vi "HW initialize hardware command.vi"(8 "error in (no error)":errorcluster, 10 "mode":T1, 11 "mmWave instrument in":refnum<class "mmWave instrument.lvclass">) -> (0 "error out":errorcluster, 3 "mmWave instrument out":refnum<class "mmWave instrument.lvclass">)   [LabVIEW 2019, in "HW Control.lvlib"]
uses:
  HW Control.lvlib
  SubVIs/mmWave instrument_class/mmWave instrument.lvclass
  SubVIs/mmWave instrument_class/Instrument mode.ctl
  SubVIs/mmWave instrument_class/Instrument state.ctl
  <vilib>/event_ctls.llb/usereventprio.ctl
  HW GV.vi
  Log/Log.lvlib
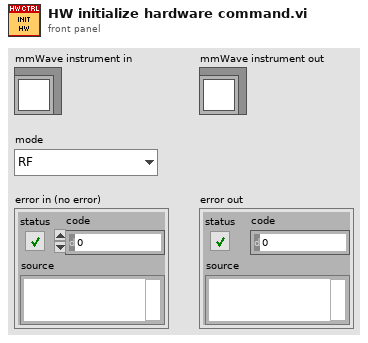
[diagram p1: front panel]
types:
  T1 = typedef "mmWave instrument.lvclass/Instrument mode.ctl" = enum16{"RF", "IF", "BB"}
  T2 = typedef "mmWave instrument.lvclass/Instrument state.ctl" = enum16{"Off", "Initialization", "Configuration", "Running", "Calibration"}
  T3 = typedef "usereventprio.ctl" = enum32{"high priority", "normal priority"}
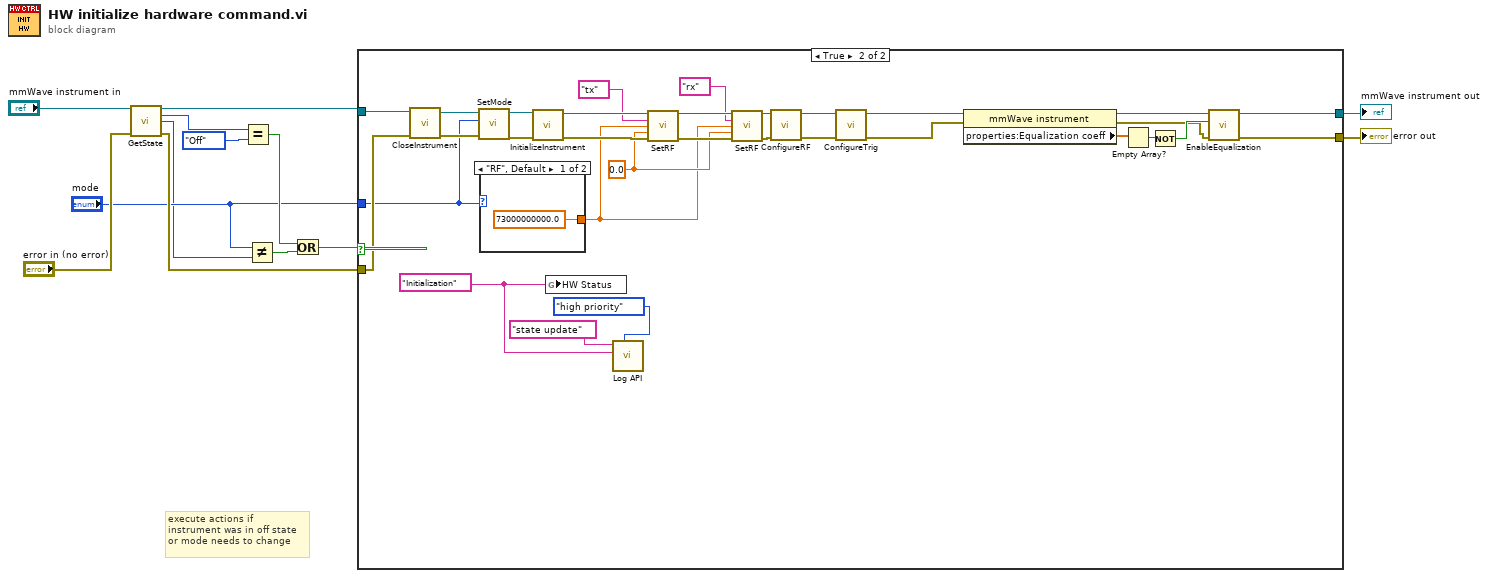
[diagram p0: block diagram]
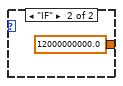
[diagram p3: hidden frame]
diagram:
  # "execute actions if\ninstrument was in off state\nor mode needs to change"
  n1 = call-dynamic "GetState.vi"("reference in"="mmWave instrument in", "error in (no error)"="error in (no error)") -> ("reference out"=w9:refnum<class "mmWave instrument.lvclass">, "state"=w2:T2, "mode"=w4:T1, "error out"=w11:errorcluster)  [unwired: 9 in, 1 out]
  n2 = Equal?(x=w2, y=Instrument_state."Off" ("x")) -> (x = y?=w7:bool)
  n3 = Not Equal?(x="mode", y=w4) -> (x != y?=w6:bool)
  n4 = Or(x=w7, y=w6) -> (x .or. y?=w8:bool)
  n5 = case shown="True" w8 {
    tunnel: w11 -> [w15 w40]
    tunnel: [w15 w20] -> w12
    tunnel: w9 -> [w14 w39]
    tunnel: "mode" -> [_ w27]
    tunnel: [w14 w25] -> w13
    frame False {
      # "no change needed"
    }
    frame True {
      w33 = 0.0 ("Gain")
      w38 = "Initialization" ("HW Status")
      n6 = call-dynamic "CloseInstrument.vi"("error in (no error)"=w40, "reference in"=w39) -> ("error out"=w45:errorcluster, "reference out"=w46:refnum<class "mmWave instrument.lvclass">)  [unwired: 8 in]
      n7 = call-dynamic "SetMode.vi"("error in (no error)"=w45, "instr mode"=w27, "reference in"=w46) -> ("error out"=w44:errorcluster, "reference out"=w43:refnum<class "mmWave instrument.lvclass">)  [unwired: 7 in]
      n8 = case shown="\"RF\", Default" w27 {
        tunnel: [73000000000.0 ("Frequency") 12000000000.0 ("Frequency")] -> w32
        frame "RF", Default {
        }
        frame "IF" {
        }
      }
      n9 = call-dynamic "InitializeInstrument.vi"("error in (no error)"=w44, "reference in"=w43) -> ("error out"=w36:errorcluster, "reference out"=w37:refnum<class "mmWave instrument.lvclass">)  [unwired: 8 in]
      n10 = global write "HW GV.vi" "HW Status"(w38) -> ()
      n11 = call "Log API.vi"("priority (normal)"=usereventprio."high priority", "data"=w38, "message"="state update") -> ()  [unwired: 8 in, 1 out]
      n12 = call-dynamic "SetRF.vi"("reference in"=w37, "Port"="tx", "Frequency"=w32, "Gain"=w33, "error in (no error)"=w36) -> ("reference out"=w35:refnum<class "mmWave instrument.lvclass">, "error out"=w34:errorcluster)  [unwired: 9 in]
      n13 = call-dynamic "SetRF.vi"("reference in"=w35, "Port"="rx", "Frequency"=w32, "Gain"=w33, "error in (no error)"=w34) -> ("reference out"=w29:refnum<class "mmWave instrument.lvclass">, "error out"=w28:errorcluster)  [unwired: 9 in]
      n14 = call-dynamic "ConfigureRF.vi"("error in (no error)"=w28, "reference in"=w29) -> ("error out"=w18:errorcluster, "reference out"=w19:refnum<class "mmWave instrument.lvclass">)  [unwired: 8 in]
      n15 = call-dynamic "ConfigureTrig.vi"("error in (no error)"=w18, "reference in"=w19) -> ("error out"=w16:errorcluster, "reference out"=w17:refnum<class "mmWave instrument.lvclass">)  [unwired: 8 in]
      n16 = property class="mmWave instrument"(reference=w17, error in=w16) -> (reference out=w26:refnum<class "mmWave instrument.lvclass">, error out=w21:errorcluster, "properties:Equalization coeff"=w24:cdb[])
      n17 = Empty Array?(array=w24) -> (empty?=w23:bool)
      n18 = Not(x=w23) -> (.not. x?=w22:bool)
      n19 = call-dynamic "EnableEqualization.vi"("error in (no error)"=w21, "Enable/Disable"=w22, "reference in"=w26) -> ("error out"=w20:errorcluster, "reference out"=w25:refnum<class "mmWave instrument.lvclass">)  [unwired: 7 in]
    }
  }
  "mmWave instrument out" <- w13
  "error out" <- w12
